vi "sv_Convert THD Results.vi"(0 "Magnitudes":cluster{"X":dbl[], "Y":dbl[]}[][](array[cluster]) {"X" format="%.2f"; "Y" format="%.2f"}, 1 "acquisition sample rate [Hz]":dbl, 9 "magnitudes info":T4[](array[typedef]) {"x-axis units" items=["Time (s)"=0, "Frequency-CB (Hz)"=1, "Frequency-CPB (Hz)"=1248, "Frequency-Arbitrary (Hz)"=2357, "Quefrency (s)"=2, "Revolutions (rev)"=3, "Order"=4, "Speed (RPM)"=11, "Speed (rad/s)"=21, "Index"=65535]; "weighting filter" items=["Linear", "A-weighting", "B-weighting", "C-weighting", "ITU-R 468-4", "Dolby", "CCITT", "C-message", "Wb", "Wc", "Wd", "We", "Wf", "Wh", "Wj", "Wk", "Wm", "AES17 20 kHz lowpass", "AES17 40 kHz lowpass", "AES17 20 kHz highpass", "AES17 40 kHz highpass"]; "dB reference [EU]" format="%.2f"; "engineering units" items=["custom..."=0, "V"=1, "A"=21, "C"=30, "pC"=31, "s"=32, "-"=29, "Pa"=2, "N"=20, "g"=3, "m/s^2"=4, "m/s"=5, "m"=6, "mm/s"=12, "mm"=13, "micron/s"=14, "micron"=15, "in/s^2"=7, "in/s"=8, "in"=9, "mil/s"=10, "mil"=11, "rad/s^2"=16, "rad/s"=17, "rad"=18, "deg/s^2"=26, "deg/s"=27, "deg"=28, "RPM"=22, "cycle/s^2"=23, "Hz"=24, "cycle"=25, "strain"=19]; "spectral info"."window" items=["None "=0, "Hanning"=1, "Hamming"=2, "Blackman-Harris"=3, "Exact Blackman"=4, "Blackman"=5, "Flat Top"=6, "4 Term B-Harris "=7, "7 Term B-Harris"=8, "Low Sidelobe"=9, "Force - Exponential"=10, "Gaussian"=62]}, 11 "harmonics to visualize":i32[](array[numeric]), 12 "desired units":T3) -> (3 "unit labels":T2(array[cluster]), 4 "THD":cluster{"frequency":dbl[], "amplitude":dbl[]}[](array[cluster]) {"amplitude" format="%.2f"; "frequency" format="%.2f"}, 6 "harmonic components":T1(array[cluster]))   [LabVIEW 2017, in "SoundVib_ContSweptSine.lvlib"]
uses:
  <vilib>/addons/Sound and Vibration/svt_Continuous Swept Sine/SoundVib_ContSweptSine.lvlib
  <vilib>/addons/_NISVFA/_Shared subVIs/Controls/svc_Spectrum Info.ctl
  <vilib>/addons/_NISVFA/_Shared subVIs/Controls/svc_X-Axis Units.ctl
  <vilib>/addons/_NISVFA/_Shared subVIs/Controls/svc_Spectrum Type.ctl
  <vilib>/addons/_NISVFA/_Shared subVIs/Controls/svc_Engineering Units Text Ring.ctl
  <vilib>/addons/_NISVFA/_Shared subVIs/Controls/svc_Weighting Filter Text Ring.ctl
  <vilib>/addons/_NISVFA/_Shared subVIs/Controls/svc_Complimentary Spectrum Units.ctl
  <vilib>/addons/Sound and Vibration/svt_Distortion/SoundVib_Distortion.lvlib
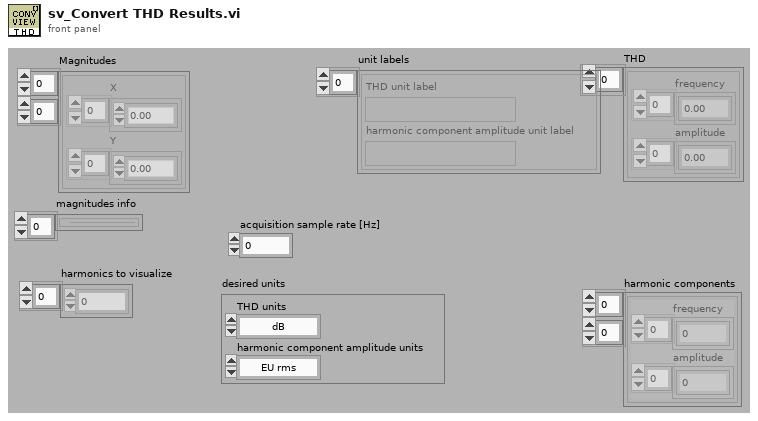
[diagram p1: front panel]
types:
  T1 = cluster{"frequency":dbl[], "amplitude":dbl[]}[][]
  T2 = cluster{"THD unit label":string, "harmonic component amplitude unit label":string}[]
  T3 = cluster{"THD units":enum16{"dB", "linear ratio", "%"}, "harmonic component amplitude units":enum16{"EU rms", "EU peak", "EU peak-peak", "dB ref fund"}}
  T4 = typedef "svc_Spectrum Info.ctl" = cluster{"channel name":string, "description":string, "x-axis units":T5, "spectral info":cluster{"spectrum type":T6, "linear/dB":enum16{"linear", "dB"}, "window":u16, "window size":i32, "FFT size":i32}, "engineering units":T7, "custom label":string, "dB reference [EU]":dbl, "peak units":enum16{"rms", "peak", "peak-peak"}, "weighting filter":T8, "spectral density?":bool, "unit label":string, "spectrum skewed?":bool, "complimentary spectrum units":T9}
  T5 = typedef "svc_X-Axis Units.ctl" = u16
  T6 = typedef "svc_Spectrum Type.ctl" = enum16{"FFT Spectrum [complex]", "Amplitude [Magnitude]", "Power [Magnitude^2]", "Cross Spectrum [complex]", "Frequency Response [Complex]"}
  T7 = typedef "svc_Engineering Units Text Ring.ctl" = u16
  T8 = typedef "svc_Weighting Filter Text Ring.ctl" = u16
  T9 = typedef "svc_Complimentary Spectrum Units.ctl" = enum16{"none", "radians", "degrees", "cycles", "imaginary"}
  T10 = enum16{"EU rms", "EU peak", "EU peak-peak", "dB ref fund"}
  T11 = cluster{"unit label":string, "unit label":string}
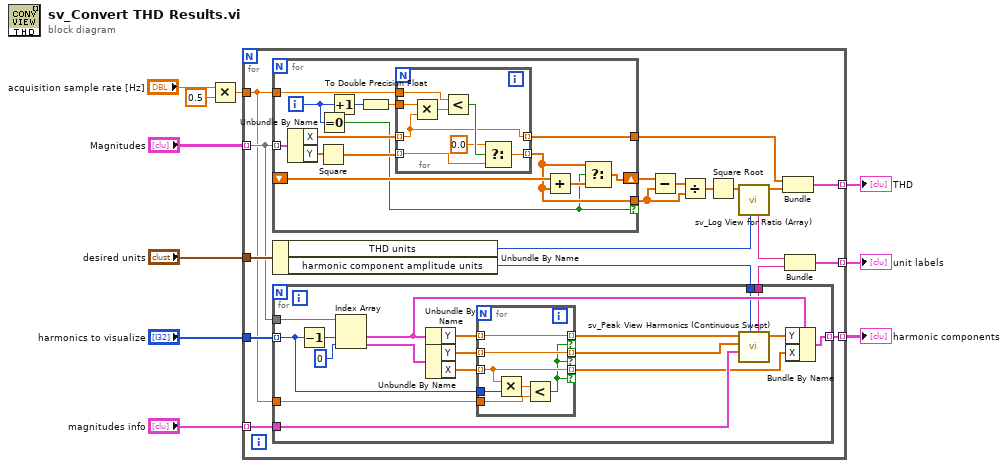
[diagram p0: block diagram]
diagram:
  n1 = Multiply(x="acquisition sample rate [Hz]", y=0.5) -> (x*y=w6:dbl)
  n2 = for {
    tunnel: "Magnitudes" -> [w18] mode=indexing
    tunnel: [w28] -> w9 mode=indexing
    tunnel: w6 -> [w11]
    tunnel: "desired units" -> [w19]
    tunnel: "magnitudes info" -> [w17] mode=indexing
    tunnel: "harmonics to visualize" -> [w16]
    tunnel: [w13] -> w2 mode=indexing
    tunnel: [w12] -> w1 mode=indexing
    n3 = for {
      tunnel: w18 -> [w68] mode=indexing
      tunnel: [w61] -> w29
      tunnel: [w59] -> w24 if=w56
      shift-right: [w64] -> w26
      shift-left: _ -> [w66]
      tunnel: w11 -> [w63]
      i -> [w58]
      n4 = Unbundle By Name(w68) -> ("X"=w62:dbl[], "Y"=w67:dbl[])
      n5 = Square(x=w67) -> (x^2=w60:dbl[])
      n6 = Equal To 0?(x=w58) -> (x = 0?=w56:bool)
      n7 = Increment(x=w58) -> (x+1=w55:i32)
      n8 = To Double Precision Float(number=w55) -> (double precision float=w57:dbl)
      n9 = for {
        tunnel: w63 -> [w76]
        tunnel: w62 -> [w69] mode=indexing
        tunnel: [w69] -> w61 mode=indexing
        tunnel: w60 -> [w74] mode=indexing
        tunnel: [w72] -> w59 mode=indexing
        tunnel: w57 -> [w71]
        n10 = Multiply(x=w71, y=w69) -> (x*y=w70:dbl)
        n11 = Less?(x=w76, y=w70) -> (x < y?=w75:bool)
        n12 = Select(t=0.0, s=w75, f=w74) -> (s? t:f=w72:dbl)
      }
      n13 = Add(x=w66, y=w59) -> (x+y=w65:dbl[])
      n14 = Select(t=w59, s=w56, f=w65) -> (s? t:f=w64:dbl[])
    }
    n15 = Unbundle By Name(w19) -> ("THD units"=w15:enum16{"dB", "linear ratio", "%"}, "harmonic component amplitude units"=w21:T10)
    n16 = for {
      tunnel: w16 -> [w37] mode=indexing
      tunnel: w18 -> [w46]
      tunnel: [w44] -> w12 mode=indexing
      tunnel: w17 -> [w43]
      tunnel: [w41] -> w20
      tunnel: w21 -> [w40]
      tunnel: w11 -> [w36]
      n17 = Decrement(x=w37) -> (x-1=w47:i32)
      n18 = Index Array(array=w46, index #1=w47, index #2=0 ("index")) -> (element #1=w45:cluster{"X":dbl[], "Y":dbl[]}, element #2=w38:cluster{"X":dbl[], "Y":dbl[]})
      n19 = Unbundle By Name(w45) -> ("Y"=w35:dbl[])
      n20 = Unbundle By Name(w38) -> ("Y"=w34:dbl[], "X"=w31:dbl[])
      n21 = for {
        tunnel: w37 -> [w53]
        tunnel: w36 -> [w52]
        tunnel: w35 -> [w51] mode=indexing
        tunnel: w34 -> [w50] mode=indexing
        tunnel: [w51] -> w32 mode=indexing if=w48
        tunnel: [w50] -> w33 mode=indexing if=w48
        tunnel: w31 -> [w49] mode=indexing
        tunnel: [w49] -> w30 mode=indexing if=w48
        n22 = Multiply(x=w49, y=w53) -> (x*y=w54:dbl)
        n23 = Less?(x=w54, y=w52) -> (x < y?=w48:bool)
      }
      n24 = call <vilib>:"sv_Peak View Harmonics (Continuous Swept).vi"("harmonic units"=w40, "spectrum info"=w43, "fundamental amplitude [EU rms]"=w33, "harmonic amplitudes [EU rms]"=w32) -> ("converted harmonic amplitudes"=w42:dbl[], "unit label"=w41:string)  [unwired: 5 in, 1 out]
      n25 = Bundle By Name(cluster=w45, "Y"=w42, "X"=w30) -> (w44:cluster{"X":dbl[], "Y":dbl[]})
    }
    n26 = Subtract(x=w26, y=w24) -> (x-y=w25:dbl[])
    n27 = Divide(x=w25, y=w24) -> (x/y=w23:dbl[])
    n28 = Square Root(x=w23) -> (sqrt(x)=w22:dbl[])
    n29 = call <vilib>:"sv_Log View for Ratio (Array).vi"("ratio units"=w15, "linear ratio"=w22) -> ("converted ratio"=w27:dbl[], "unit label"=w14:string)  [unwired: 7 in, 1 out]
    n30 = Bundle(w29, "converted ratio"=w27) -> (w28:cluster{dbl[], "converted ratio":dbl[]})  [unwired: 1 in]
    n31 = Bundle("unit label"=w14, "unit label"=w20) -> (w13:T11)  [unwired: 1 in]
  }
  "THD" <- w9
  "unit labels" <- w2
  "harmonic components" <- w1
